vi "Configuration Files.vi"(8 "error in":errorcluster, 11 "Node Ptr":T1 format="%.0x") -> (0 "error out":errorcluster)   [LabVIEW 2023, in "Ballard MIL-STD-1553 System Explorer.lvlib" / "Implementation.lvlib"]
uses:
  Implementation.lvlib
  <vilib>/NI VeriStand/Custom Device API/Custom Device Item Ref.ctl
  <vilib>/NI VeriStand/Custom Device API/Custom Device API.lvlib
  Scripting/Ballard MIL-STD-1553 Scripting.lvlib
  Refresh/Refresh.lvlib
panel:
  in  "Create Tx/Rx Folders for Subaddresses?":bool=TRUE
  in  "refresh":bool
  in  "parameter config file path":path caption="Parameter Configuration File Path"
  in  "HW config file path":path caption="Hardware Configuration File Path"
  in  "SHDocVw.IWebBrowser":refnum<k7>(container)
  in  "General Header":cluster{"Section Name":string}={"Section Name"="Ballard MIL-STD-1553 - Configuration Files"}
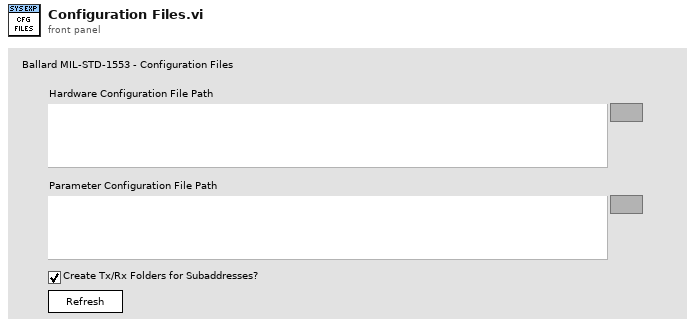
[diagram p1: front panel]
types:
  T1 = typedef "Custom Device API.lvlib/Custom Device Item Ref.ctl" = u64
  T2 = typedef "Custom Device API.lvlib/Custom Device Commands.ctl" = enum16{"Default", "Item renamed", "Shutdown", "Dynamic button pressed"}
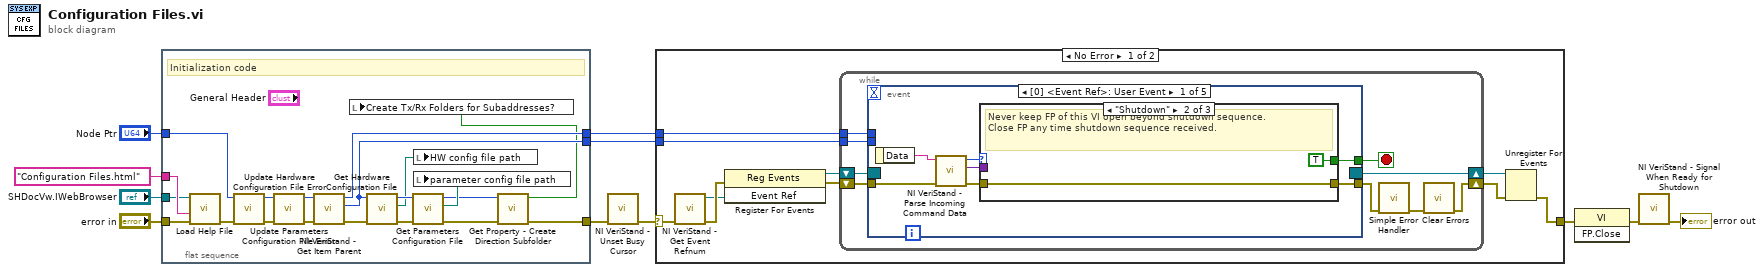
[diagram p0: block diagram]
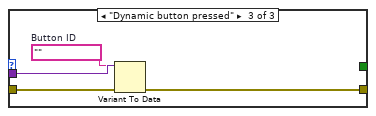
[diagram p3: hidden frame]
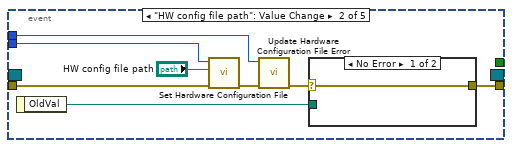
[diagram p4: hidden frame]
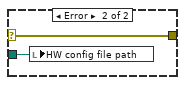
[diagram p5: hidden frame]
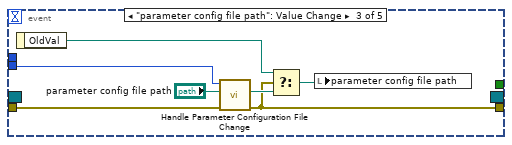
[diagram p6: hidden frame]
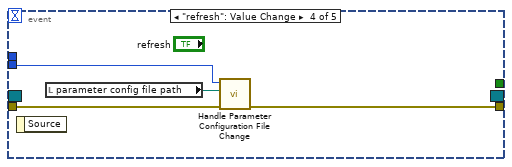
[diagram p7: hidden frame]
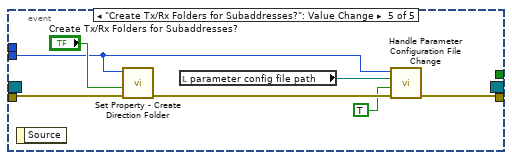
[diagram p8: hidden frame]
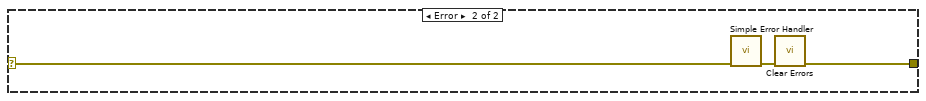
[diagram p9: hidden frame]
diagram:
  n1 = flat-sequence "Initialization code" {
    tunnel: "error in" -> [w31]
    tunnel: "Node Ptr" -> [w18]
    tunnel: [w14] -> w7
    tunnel: "SHDocVw.IWebBrowser" -> [w29]
    tunnel: "Configuration Files.html" ("CD_CHM_Section") -> [w30]
    tunnel: [w23] -> w2
    tunnel: [w22] -> w1
    frame #0 {
      # "Initialization code"
      n2 = call "Load Help File.vi"("error in (no error)"=w31, "HTML File to Load"=w30, "Browser"=w29) -> ("error out"=w19:errorcluster)  [unwired: 8 in]
      n3 = call "Update Hardware Configuration File Error.vi"("error in"=w19, "configuration files ref in"=w18) -> ("error out"=w20:errorcluster, "configuration files ref out"=w21:T1)  [unwired: 8 in]
      n4 = call "Update Parameters Configuration File Error.vi"("error in"=w20, "configuration files ref in"=w21) -> ("error out"=w17:errorcluster, "configuration files ref out"=w16:T1)  [unwired: 8 in]
      n5 = call <vilib>:"NI VeriStand - Get Item Parent.vi"("error in (no error)"=w17, "Item Ref in"=w16) -> ("error out"=w28:errorcluster, "Parent Ref"=w23:T1, "Item Ref out"=w22:T1)  [unwired: 6 in, 1 out]
      n6 = call "Get Hardware Configuration File.vi"("error in"=w28, "Ballard MIL-STD 1553 custom device in"=w23) -> ("error out"=w26:errorcluster, "hardware configuration file"=w25:path, "Ballard MIL_STD 1553 custom device out"=w27:T1)  [unwired: 6 in, 1 out]
      n7 = call "Get Parameters Configuration File.vi"("error in"=w26, "Ballard MIL-STD 1553 custom device in"=w27) -> ("error out"=w15:errorcluster, "parameters configuration file"=w24:path, "Ballard MIL-STD 1553 custom device out"=w13:T1)  [unwired: 6 in, 1 out]
      n8 = local write "HW config file path"(w25) -> ()
      n9 = local write "parameter config file path"(w24) -> ()
      n10 = call "Get Property - Create Direction Subfolder.vi"("error in"=w15, "custom device"=w13) -> ("error out"=w14:errorcluster, "Value"=w12:bool)  [unwired: 8 in]
      n11 = local write "Create Tx/Rx Folders for Subaddresses?"(w12) -> ()
    }
  }
  n12 = call <vilib>:"NI VeriStand - Unset Busy Cursor.vi"("error in (no error)"=w7) -> ("error out"=w6:errorcluster)  [unwired: 10 out]
  n13 = case shown="No Error" w6 {
    selector: w6 -> [w34 w96]
    tunnel: [w38 w94] -> w11
    tunnel: w2 -> [w33 _]
    tunnel: w1 -> [w32 _]
    frame No Error {
      n14 = call <vilib>:"NI VeriStand - Get Event Refnum.vi"("error in (no error)"=w34) -> ("error out"=w41:errorcluster, "Event Ref"=w37:refnum<user-event>)  [unwired: 9 out]
      n15 = register-events(error in=w41, w37) -> (reference out=w35:refnum<event-registration>, error out=w36:errorcluster)  [unwired: 1 in]
      n16 = while {
        shift-right: [w44] -> w39
        shift-left: w36 -> [w49]
        shift-right: [w50] -> w40
        shift-left: w35 -> [w48]
        tunnel: w33 -> [w43]
        tunnel: w32 -> [w42]
        stop <- w47 stop-if-true
        n17 = event shown="[0] <Event Ref>: User Event" {
          selector: w48 -> [_ _ _ _ _]
          dyn-events: [_ _ _ _ _] -> w50
          timeout: _ -> [_ _ _ _ _]
          tunnel: w49 -> [w57 w72 w82 w85 w93]
          tunnel: [w54 _ _ _ _] -> w47
          tunnel: [w53 w70 w78 w86 w89] -> w46
          tunnel: w43 -> [_ w68 w81 w84 w88]
          tunnel: w42 -> [_ w65 _ _ _]
          event User Event {
            n18 = event-data() -> ("Data"=w51:string)  [unwired: 1 out]
            n19 = call <vilib>:"NI VeriStand - Parse Incoming Command Data.vi"("error in (no error)"=w57, "Incoming data"=w51) -> ("error out"=w56:errorcluster, "Outgoing data"=w52:variant, "Action"=w55:T2)  [unwired: 7 out]
            n20 = case shown="\"Shutdown\"" w55 {
              tunnel: w56 -> [w58 w59 w64]
              tunnel: [_ TRUE _] -> w54
              tunnel: [w58 w59 w61] -> w53
              tunnel: w52 -> [_ _ w63]
              frame Default {
                # "Ignore"
              }
              frame "Shutdown" {
                # "Never keep FP of this VI open beyond shutdown sequence.\nClose FP any time shutdown sequence received."
              }
              frame "Dynamic button pressed" {
                w62 = ""  # Button ID
                n21 = Variant To Data(error in=w64, type=w62, Variant=w63) -> (error out=w61:errorcluster)  [unwired: 1 out]
              }
            }
          }
          event "HW config file path": Value Change {
            n22 = event-data() -> ("OldVal"=w69:path)  [unwired: 1 out]
            n23 = call "Set Hardware Configuration File.vi"("error in"=w72, "hardware configuration file path"="HW config file path", "Ballard MIL-STD 1553 custom device in"=w68) -> ("error out"=w67:errorcluster)  [unwired: 7 in, 1 out]
            n24 = call "Update Hardware Configuration File Error.vi"("error in"=w67, "configuration files ref in"=w65) -> ("error out"=w66:errorcluster)  [unwired: 8 in, 1 out]
            n25 = case shown="No Error" w66 {
              selector: w66 -> [w73 w75]
              tunnel: [w73 w75] -> w70
              tunnel: w69 -> [_ w74]
              frame No Error {
              }
              frame Error {
                n26 = local write "HW config file path"(w74) -> ()
              }
            }
          }
          event "parameter config file path": Value Change {
            n27 = event-data() -> ("OldVal"=w77:path)  [unwired: 1 out]
            n28 = call "Handle Parameter Configuration File Change.vi"("error in"=w82, "new parameter configuration file path"="parameter config file path", "Ballard MIL-STD-1553 custom device in"=w81) -> ("error out"=w78:errorcluster, "parameters configuration file out"=w79:path)  [unwired: 6 in, 1 out]
            n29 = Select(t=w77, s=w78, f=w79) -> (s? t:f=w76:path)
            n30 = local write "parameter config file path"(w76) -> ()
          }
          event "refresh": Value Change {
            n31 = event-data() -> ()  [unwired: 2 out]
            n32 = local read "parameter config file path"() -> (w83:path)
            n33 = call "Handle Parameter Configuration File Change.vi"("error in"=w85, "new parameter configuration file path"=w83, "Ballard MIL-STD-1553 custom device in"=w84) -> ("error out"=w86:errorcluster)  [unwired: 6 in, 2 out]
          }
          event "Create Tx/Rx Folders for Subaddresses?": Value Change {
            n34 = event-data() -> ()  [unwired: 2 out]
            n35 = call "Set Property - Create Direction Folder.vi"("error in"=w93, "create Tx/Rx folders for subaddresses?"="Create Tx/Rx Folders for Subaddresses?", "custom device"=w88) -> ("error out"=w91:errorcluster)  [unwired: 7 in, 1 out]
            n36 = local read "parameter config file path"() -> (w90:path)
            n37 = call "Handle Parameter Configuration File Change.vi"("error in"=w91, "create Tx/Rx folders for subaddresses value change?"=TRUE, "new parameter configuration file path"=w90, "Ballard MIL-STD-1553 custom device in"=w88) -> ("error out"=w89:errorcluster)  [unwired: 5 in, 2 out]
          }
        }
        n38 = call <vilib>:"Simple Error Handler.vi"("error in (no error)"=w46) -> ("error out"=w45:errorcluster)  [unwired: 1 in, 7 out]
        n39 = call <vilib>:"Clear Errors.vi"("error in (no error)"=w45) -> ("error out"=w44:errorcluster)  [unwired: 1 in, 5 out]
      }
      n40 = Unregister For Events(event registration refnum=w40, error in=w39) -> (error out=w38:errorcluster)
    }
    frame Error {
      n41 = call <vilib>:"Simple Error Handler.vi"("error in (no error)"=w96) -> ("error out"=w95:errorcluster)  [unwired: 1 in, 7 out]
      n42 = call <vilib>:"Clear Errors.vi"("error in (no error)"=w95) -> ("error out"=w94:errorcluster)  [unwired: 1 in, 5 out]
    }
  }
  n43 = invoke class="VI" method="FP.Close"(error in=w11) -> (error out=w10:errorcluster)  [unwired: 2 in, 2 out]
  n44 = call <vilib>:"NI VeriStand - Signal When Ready for Shutdown.vi"("error in (no error)"=w10) -> ("error out"=→"error out":errorcluster)  [unwired: 10 out]
